vi "PostScanAction.vi"(0 "Device en entrée":refnum<class "Spex.lvclass"> caption="DNL_LabVIEW Object in", 5 "AcqComp":bool, 7 "ScanDev":bool caption="AcqComp", 11 "error in (no error)":errorcluster caption="entrée d'erreur (pas d'erreur)") -> (4 "Device en sortie":refnum<class "Spex.lvclass"> caption="DNL_LabVIEW Object out", 6 "PostScanString":string, 15 "error out":errorcluster caption="sortie d'erreur")   [LabVIEW 2019, in "Spex.lvclass"]
uses:
  Spex.lvclass
  C:/Programmes Labview/LabscanV1A/DevicesClass/BaseDevice/BaseDevice.lvclass
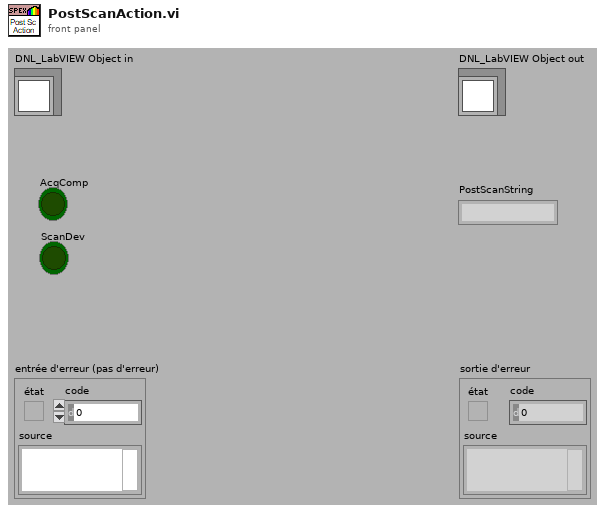
[diagram p1: front panel]
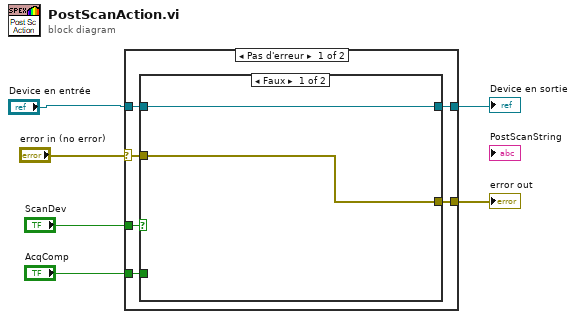
[diagram p0: block diagram]
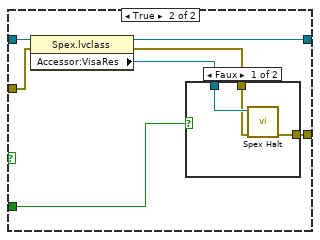
[diagram p2: hidden frame]
diagram:
  n1 = case shown="Pas d'erreur" "error in (no error)" {
    selector: "error in (no error)" -> [w11 w26]
    tunnel: "Device en entrée" -> [w12 w27]
    tunnel: [w10 w27] -> w4
    tunnel: [w9 w26] -> w3
    tunnel: "AcqComp" -> [w8 _]
    tunnel: "ScanDev" -> [w7 _]
    frame No Error {
      n2 = case shown="Faux" w7 {
        tunnel: w12 -> [w14 w21]
        tunnel: w11 -> [w13 w20]
        tunnel: [w14 w19] -> w10
        tunnel: [w13 w16] -> w9
        tunnel: w8 -> [_ w15]
        frame False {
        }
        frame True {
          n3 = property class="Spex.lvclass"(reference=w21, error in=w20) -> (reference out=w19:refnum<class "Spex.lvclass">, error out=w17:errorcluster, "Accessor:VisaRes"=w18:refnum<visa-resource-name>)
          n4 = case shown="Faux" w15 {
            tunnel: w18 -> [w24 _]
            tunnel: w17 -> [w23 w25]
            tunnel: [w22 w25] -> w16
            frame False {
              n5 = call <userlib>:"Spex Halt.vi"("error in"=w23, "Spex Port"=w24) -> ("error out"=w22:errorcluster)  [unwired: 8 in, 1 out]
            }
            frame True {
            }
          }
        }
      }
    }
    frame Error {
    }
  }
  "error out" <- w3
  "Device en sortie" <- w4
